vi "Test ISO8601 DateTime Strings.vi"(8 "error in":errorcluster) -> (0 "error out":errorcluster)   [LabVIEW 2013]
uses:
  <vilib>/addons/_JKI Toolkits/Caraya/classes/Test/Test.lvclass
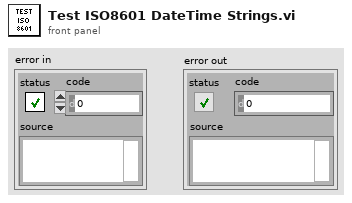
[diagram p1: front panel]
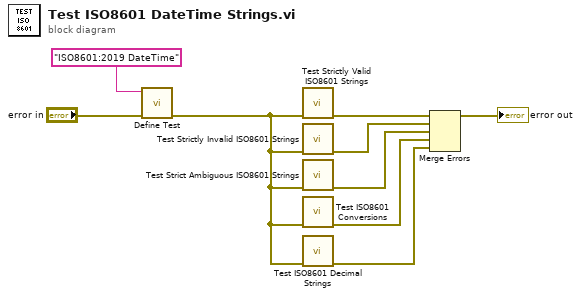
[diagram p0: block diagram]
diagram:
  n1 = call <vilib>:"Define Test.vi"("error in (no error)"="error in", "Label (VI Title)"="ISO8601:2019 DateTime") -> ("error out"=w2:errorcluster)  [unwired: 8 in, 1 out]
  n2 = call "Test Strictly Valid ISO8601 Strings.vi"("error in (no error)"=w2) -> ("error out"=w4:errorcluster)  [unwired: 10 in]
  n3 = call "Test Strictly Invalid ISO8601 Strings.vi"("error in (no error)"=w2) -> ("error out"=w5:errorcluster)  [unwired: 10 in]
  n4 = call "Test Strict Ambiguous ISO8601 Strings.vi"("error in (no error)"=w2) -> ("error out"=w6:errorcluster)  [unwired: 10 in]
  n5 = call "Test ISO8601 Conversions.vi"("error in (no error)"=w2) -> ("error out"=w3:errorcluster)  [unwired: 10 in]
  n6 = call "Test ISO8601 Decimal Strings.vi"("error in (no error)"=w2) -> ("error out"=w1:errorcluster)  [unwired: 10 in]
  n7 = Merge Errors(w4, w5, w6, w3, w1) -> (→"error out":errorcluster)
